vi "G# - DependencyInjectionUsingGenericCreate.vi"() -> ()   [LabVIEW 2017]
doc: "Dependency Injection with G# Generic Create\nThis example demonstrates how the G#Object_GenericCreate.vi works. This type of implementation can be used to create a injection/plug in pattern when building architectures. Please notice that this method uses VI server and will execute the constructor as a running top-level execution VI.\n\nBy using the G# Debugger found in Tools->G# Debugger a text log can be followed showing how the objects were created and destroyed."
uses:
  MyG#SubClass_class/MyG#SubClass.lvclass
  vi.lib/addons/_AddQ/G#Object/G#Object.lvclass
panel:
  out "class path":path
  in  "control names":string[](array[string])=["MyAttribute", "MySubAttribute"]
  in  "My G#Object SubAttribute in":dbl=5.0
  in  "My G#Object Attribute in":dbl=2.0
  in  "error in (no error)":errorcluster
  out "My G#Object SubAttribute out":dbl
  out "My G#Object Attribute out":dbl
  out "class name":string
  out "error out":errorcluster
  out "OK":bool
  out "# of objects killed":i32
  # "Dependency Injection with G# Generic Create\nThis example demonstrates how the G#Object_GenericCreate.vi works. This type of implementation can be used to create a injection/plug-in\npattern when building architectures. Please notice that this method uses VI server and will execute the constructor as a running top-level execution VI.\n\nBy using the G# Debugger found in Tools->G# Debugger a text log can be followed showing how the objects were created and destroyed."
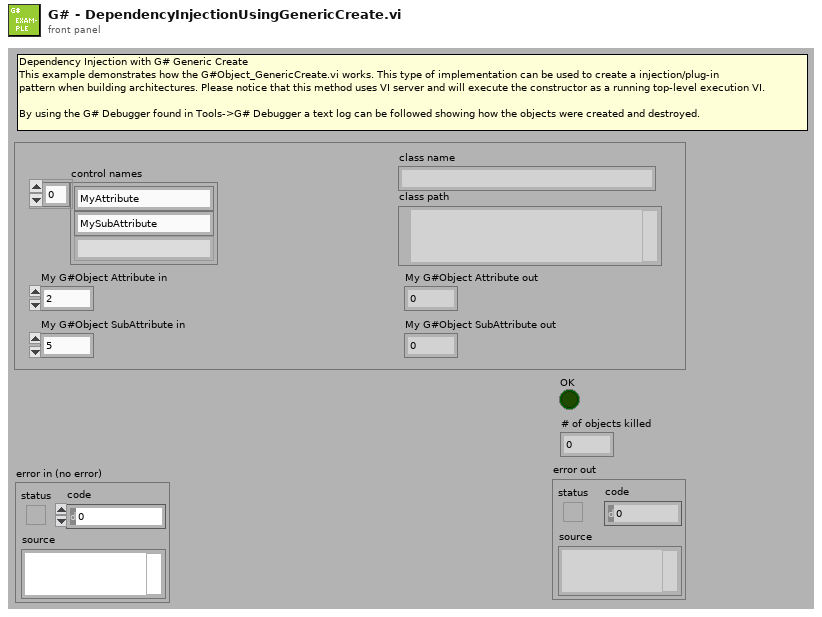
[diagram p1: front panel]
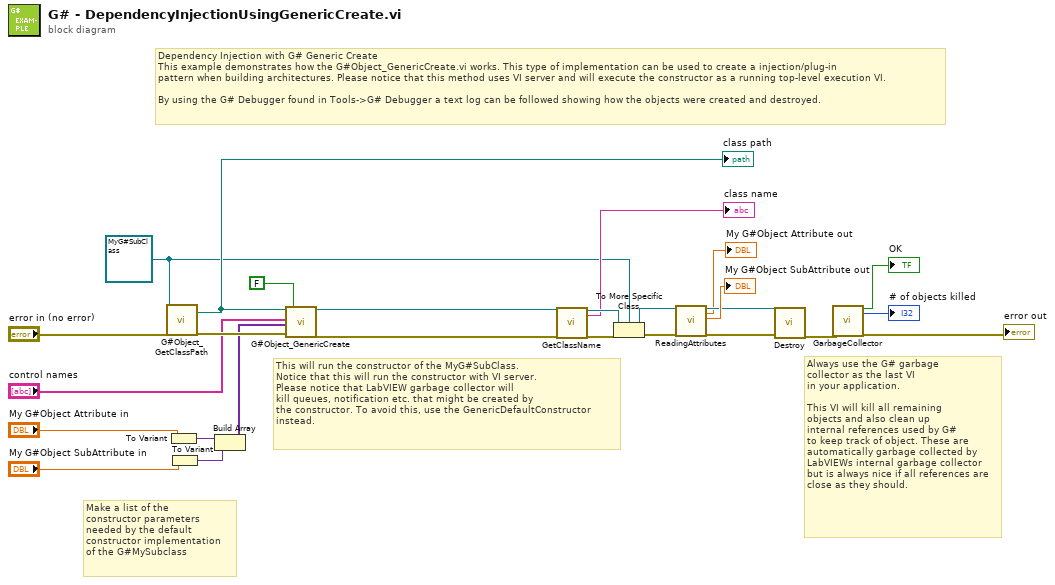
[diagram p0: block diagram]
diagram:
  w10 = refnum<class "MyG#SubClass.lvclass"> refnum ("MyG#SubClass.lvclass")
  # "Dependency Injection with G# Generic Create\nThis example demonstrates how the G#Object_GenericCreate.vi works. This type of implementation can be used to create a injection/plug-in\npattern when building architectures. Please notice that this method uses VI server and will execute the constructor as a running top-level execution VI.\n\nBy using the G# Debugger found in Tools->G# Debugger a text log can be followed showing how the objects were created and destroyed."
  # "This will run the constructor of the MyG#SubClass.\nNotice that this will run the constructor with VI server.\nPlease notice that LabVIEW garbage collector will\nkill queues, notification etc. that might be created by\nthe constructor. To avoid this, use the GenericDefaultConstructor\ninstead."
  # "Always use the G# garbage\ncollector as the last VI\nin your application.\n\nThis VI will kill all remaining\nobjects and also clean up\ninternal references used by G#\nto keep track of object. These are\nautomatically garbage collected by\nLabVIEWs internal garbage collector\nbut is always nice if all references are\nclose as they should."
  # "Make a list of the \nconstructor parameters\nneeded by the default\nconstructor implementation\nof the G#MySubclass"
  n1 = call-dynamic "G#Object_GetClassPath.vi"("reference in"=w10, "error in (no error)"="error in (no error)") -> ("class path"=w25:path, "error out"=w26:errorcluster)  [unwired: 15 in, 1 out]
  "class path" <- w25
  n2 = To Variant(anything="My G#Object Attribute in") -> (Variant=w24:variant)
  n3 = To Variant(anything="My G#Object SubAttribute in") -> (Variant=w23:variant)
  n4 = Build Array(w24, w23) -> (w20:variant[])
  n5 = call "G#Object_GenericCreate.vi"("class path"=w25, "control names"="control names", "control values"=w20, "error in (no error)"=w26, "keep constructor VI ref open? (T)"=FALSE ("keep constructor VI ref open")) -> ("reference out"=w7:refnum<class "G#Object.lvclass">, "error out"=w6:errorcluster)  [unwired: 12 in, 1 out]
  n6 = call-dynamic "GetClassName.vi"("reference in"=w7, "error in (no error)"=w6) -> ("reference out"=w17:refnum<class "G#Object.lvclass">, "class name"=→"class name":string, "error out"=w18:errorcluster)  [unwired: 13 in, 2 out]
  n7 = To More Specific Class(target class=w10, reference=w17, error in=w18) -> (specific class reference=w15:refnum<class "MyG#SubClass.lvclass">, error out=w16:errorcluster)
  n8 = call-dynamic "ReadingAttributes.vi"("reference in"=w15, "error in (no error)"=w16) -> ("reference out"=w12:refnum<class "MyG#SubClass.lvclass">, "MyAttribute"=→"My G#Object Attribute out":dbl, "MySubAttribute"=→"My G#Object SubAttribute out":dbl, "error out"=w14:errorcluster)  [unwired: 14 in]
  n9 = call-dynamic "Destroy.vi"("reference in"=w12, "error in (no error)"=w14) -> ("error out"=w4:errorcluster)  [unwired: 16 in, 1 out]
  n10 = call "GarbageCollector.vi"("error in (no error)"=w4) -> ("OK"=→"OK":bool, "# of objects killed"=→"# of objects killed":i32, "error out"=→"error out":errorcluster)  [unwired: 16 in]
